vi "22 Frequency Average (x64-2018).vi"(1 "Frequency":dynamicdata(waveform)) -> (0 "Numeric":dbl)   [LabVIEW 2017]
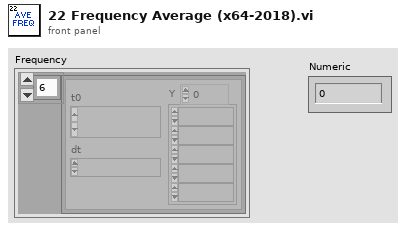
[diagram p1: front panel]
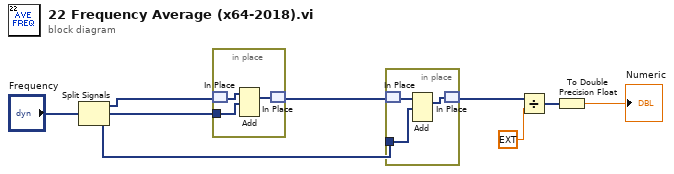
[diagram p0: block diagram]
diagram:
  n1 = Split Signals("Frequency") -> (w3:dynamicdata, w4:dynamicdata, w6:dynamicdata)  [unwired: 3 in]
  n2 = in-place {
    in-place-border: w4 -> [w11]
    n3 = in-place-match #1(w3) -> (w10:dynamicdata)
    n4 = Add(1:w11, 2:w10) -> (0:w12:dynamicdata)  [unwired: 1 in, 1 out]
    n5 = in-place-match #1(w12) -> (w5:dynamicdata)
  }
  n6 = in-place {
    in-place-border: w6 -> [w14]
    n7 = in-place-match #2(w5) -> (w13:dynamicdata)
    n8 = Add(1:w14, 2:w13) -> (0:w15:dynamicdata)  [unwired: 1 in, 1 out]
    n9 = in-place-match #2(w15) -> (w7:dynamicdata)
  }
  n10 = Divide(x=w7, y=ext 3.0) -> (x/y=w9:dynamicdata)
  n11 = To Double Precision Float(number=w9) -> (double precision float=→"Numeric":dbl)
